vi "dvp Vi Get Awb Roi.vi"(6 "pH":i32, 7 "pW":i32, 9 "pY":i32, 10 "pX":i32, 11 "handle":u32) -> (1 "pY out":i32, 2 "pX out":i32, 3 "function return":u32(ring), 4 "pH out":i32, 5 "pW out":i32)   [LabVIEW 2018, in "LabViewDVPCamera.lvlib"]
doc: "LabviewDvp2Api dvpStatus dvpViGetAwbRoi(\n dvpHandle handle, \n dvpInt32 *pX,\n dvpInt32 *pY,\n dvpInt32 *pW,\n dvpInt32 *pH);"
uses:
  LabViewDVPCamera.lvlib
  LabViewDVPCamera/LabViewDVPCamera.dll
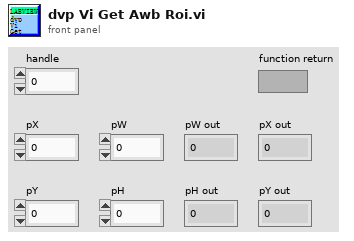
[diagram p1: front panel]
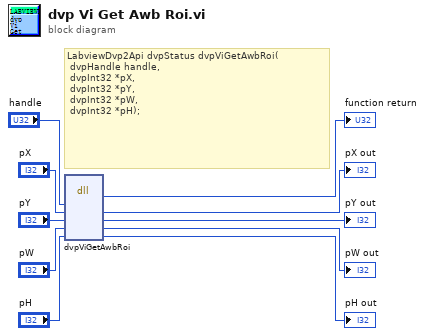
[diagram p0: block diagram]
diagram:
  # "LabviewDvp2Api dvpStatus dvpViGetAwbRoi(\n\tdvpHandle handle, \n\tdvpInt32 *pX,\n\tdvpInt32 *pY,\n\tdvpInt32 *pW,\n\tdvpInt32 *pH);"
  n1 = dll-call lib="C:/Program Files (x86)/DVP2 Labview cn 64/Sample/LabViewDVPCamera/LabViewDVPCamera.*" fn="dvpViGetAwbRoi"("handle"="handle", "pX"="pX", "pY"="pY", "pW"="pW", "pH"="pH") -> (→"function return":u32, "pX"=→"pX out":i32, "pY"=→"pY out":i32, "pW"=→"pW out":i32, "pH"=→"pH out":i32)  [unwired: 4 in, 2 out]
